vi "))Channel.vi"(6 "abort (F)":bool, 7 "This VI":refnum<vi>, 8 "element in":cluster{timestamp[], dbl[]}[](array[cluster]), 10 "channelOp":T2=enum."write", 11 "channel in":T1) -> (0 "element out":cluster{timestamp[], dbl[]}[](array[cluster]), 1 "sequence":u64, 2 "wait":refnum<k4>, 3 "channel out":T1, 4 "aborted?":bool, 5 "This VI out":refnum<vi>)   [LabVIEW 2020, in "Tag-a[.](c(a[.](stamp),a[.](dbl))).lvlib"]
uses:
  <extravilib>/ChannelInstances/Tag-a[.](c(a[.](stamp),a[.](dbl))).lvlib
  <extravilib>/ChannelInstances/Tag-a[.](c(a[.](stamp),a[.](dbl)))/ChannelOp.ctl
  <extravilib>/ChannelInstances/Tag-a[.](c(a[.](stamp),a[.](dbl)))/))Channel.ctl
  <extravilib>/ChannelInstances/Tag-a[.](c(a[.](stamp),a[.](dbl)))/TagData.lvclass
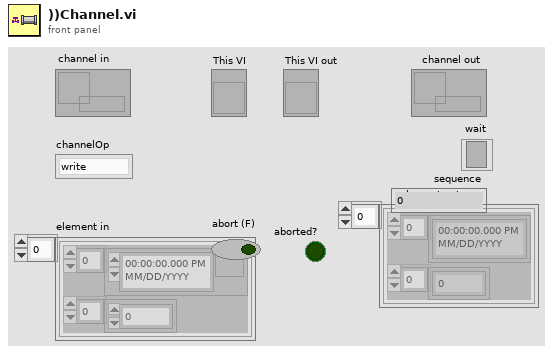
[diagram p1: front panel]
types:
  T1 = typedef "Tag-a[.](c(a[.](stamp),a[.](dbl))).lvlib/))Channel.ctl" = refnum<queue>
  T2 = typedef "Tag-a[.](c(a[.](stamp),a[.](dbl))).lvlib/ChannelOp.ctl" = enum16{"init", "write", "read", "probe"}
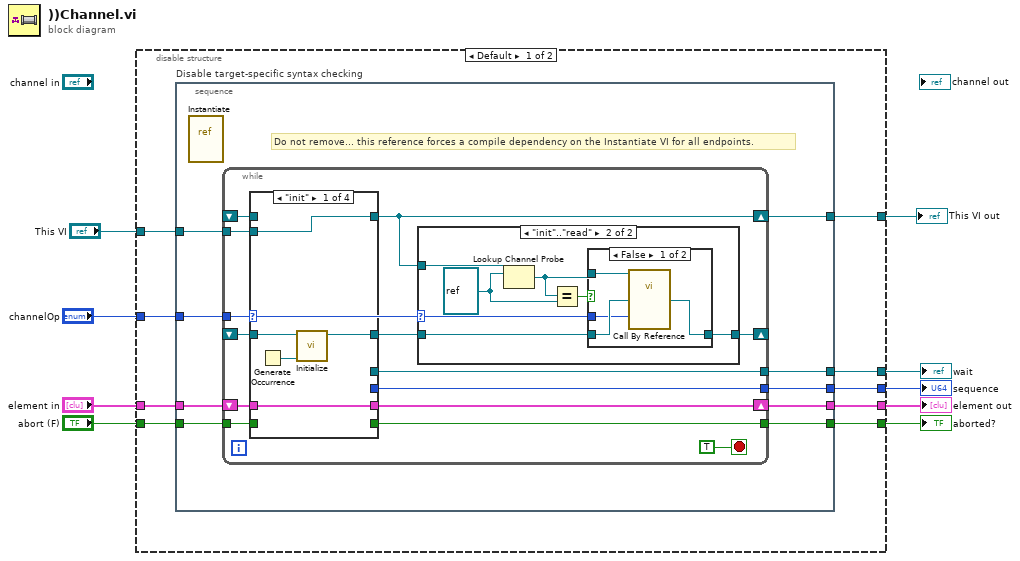
[diagram p0: block diagram]
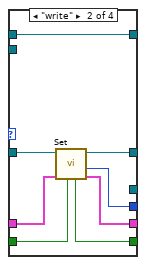
[diagram p2: hidden frame]
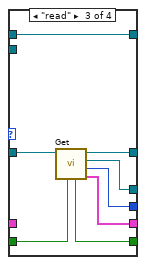
[diagram p3: hidden frame]
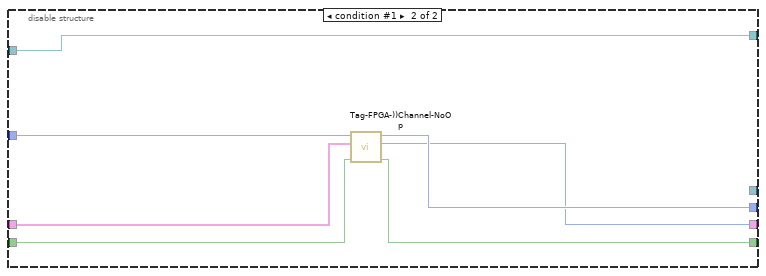
[diagram p7: hidden frame]
diagram:
  n1 = disable-structure "Conditional Disable Structure" shown="Default" {
    disable-tunnel: "channelOp" -> [w17 w85]
    disable-tunnel: "element in" -> [w18 w84]
    disable-tunnel: [w15 w83] -> w7
    disable-tunnel: [w14 w82] -> w6
    disable-tunnel: [w16 _] -> w5
    disable-tunnel: "abort (F)" -> [w13 w81]
    disable-tunnel: [w12 w80] -> w3
    disable-tunnel: "This VI" -> [w11 w79]
    disable-tunnel: [w10 w79] -> w1
    frame condition #0 (active) {
      n2 = stacked-sequence "Disable target-specific syntax checking" {
        tunnel: w18 -> [w27]
        tunnel: w17 -> [w26]
        tunnel: [w25] -> w16
        tunnel: [w24] -> w15
        tunnel: [w23] -> w14
        tunnel: w13 -> [w22]
        tunnel: [w21] -> w12
        tunnel: w11 -> [w20]
        tunnel: [w19] -> w10
        frame #0 {
          # "Do not remove... this reference forces a compile dependency on the Instantiate VI for all endpoints."
          n3 = vi-ref <extravilib>:"Instantiate.vi"() -> ()  [unwired: 1 out]
          n4 = while {
            tunnel: w26 -> [w31]
            shift-right: [w35] -> _
            shift-left: _ -> [w41]
            tunnel: [w39] -> w25
            tunnel: [w38] -> w24
            tunnel: w22 -> [w33]
            tunnel: [w32] -> w21
            shift-right: [w28] -> w19
            shift-left: _ -> [w29]
            tunnel: w20 -> [w30]
            shift-right: [w37] -> w23
            shift-left: w27 -> [w36]
            stop <- TRUE stop-if-true
            n5 = case shown="\"init\"" w31 {
              tunnel: [w46 w53 w61 w65] -> w34
              tunnel: w41 -> [w45 w54 w62 w65]
              tunnel: [_ _ w60 _] -> w39
              tunnel: [_ w51 w59 _] -> w38
              tunnel: [w42 w47 w58 w63] -> w37
              tunnel: w36 -> [w42 w52 _ w63]
              tunnel: w33 -> [_ w50 w56 _]
              tunnel: [_ w49 w57 _] -> w32
              tunnel: w30 -> [w43 _ _ _]
              tunnel: [w43 w48 w55 w64] -> w28
              tunnel: w29 -> [_ w48 w55 w64]
              frame "init" {
                n6 = Generate Occurrence() -> (w44:refnum<k4>)
                n7 = call <extravilib>:"Initialize.vi"("update"=w44, "TagData in"=w45) -> ("TagData out"=w46:refnum<class "TagData.lvclass">)  [unwired: 9 in]
              }
              frame "write" {
                n8 = call <extravilib>:"Set.vi"("abort (F)"=w50, "element"=w52, "TagData in"=w54) -> ("previous element"=w47:cluster{timestamp[], dbl[]}[], "sequence"=w51:u64, "TagData out"=w53:refnum<class "TagData.lvclass">, "aborted?"=w49:bool)  [unwired: 5 in]
              }
              frame "read" {
                n9 = call <extravilib>:"Get.vi"("abort (F)"=w56, "TagData in"=w62) -> ("element"=w58:cluster{timestamp[], dbl[]}[], "sequence"=w59:u64, "update"=w60:refnum<k4>, "TagData out"=w61:refnum<class "TagData.lvclass">, "aborted?"=w57:bool)  [unwired: 5 in]
              }
              frame "probe" {
              }
            }
            n10 = case shown="\"init\"..\"read\"" w31 {
              selector: w31 -> [_ w69]
              tunnel: w34 -> [w66 w71]
              tunnel: [w66 w70] -> w35
              tunnel: w28 -> [_ w67]
              frame Default {
              }
              frame "init".."read" {
                w68 = refnum<vi> refnum ("This VI")
                n11 = Lookup Channel Probe(0:w67, 1:w68) -> (9:w72:refnum<vi>)  [unwired: 1 in, 1 out]
                n12 = Equal?(x=w72, y=w68) -> (x = y?=w73:bool)
                n13 = case shown="False" w73 {
                  tunnel: w72 -> [w77 _]
                  tunnel: w71 -> [w76 w78]
                  tunnel: [w75 w78] -> w70
                  tunnel: w69 -> [w74 _]
                  frame False {
                    n14 = call-by-ref "?"(reference=w77, "channelOp"=w74, "tagData in"=w76) -> ("tagData out"=w75:refnum<class "TagData.lvclass">)  [unwired: 2 in, 2 out]
                  }
                  frame True {
                  }
                }
              }
            }
          }
        }
      }
    }
    frame condition #1 {
      n15 = call <extravilib>:"Tag-FPGA-))Channel-NoOp.vi"("abort (F)"=w81, "element in"=w84, "channelOp"=w85) -> ("aborted?"=w80:bool, "element out"=w82:i32, "sequence"=w83:i16)  [unwired: 6 in]
    }
  }
  "element out" <- w6
  "wait" <- w5
  "sequence" <- w7
  "aborted?" <- w3
  "This VI out" <- w1
